vi "Mode_Select.vi"(1 "Input Data":T1) -> (0 "Signal Sequence [V]":dbl[](array[numeric]))   [LabVIEW 2023]
doc: "This Simple VI is aimed at extracting the sequece of interest, depending on the enumerator \"Type of the signal\".\nInputs:\n- Cluster (Matrix of the signals, Enumerator with the required type of signal).\nOutputs:\n- Required Signal"
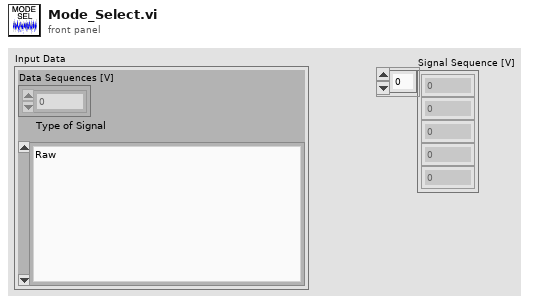
[diagram p1: front panel]
types:
  T1 = cluster{"Data Sequences [V]":dbl[][], "Type of Signal":enum16{"Raw", "Envelopped"}}
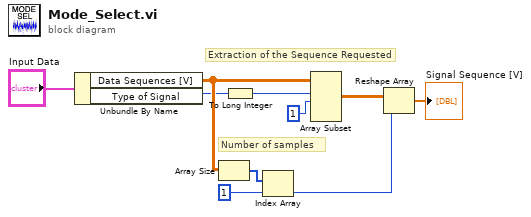
[diagram p0: block diagram]
diagram:
  # "Number of samples"
  # "Extraction of the Sequence Requested"
  n1 = Unbundle By Name("Input Data") -> ("Data Sequences [V]"=w3:dbl[][], "Type of Signal"=w1:enum16{"Raw", "Envelopped"})
  n2 = Array Size(array=w3) -> (size(s)=w5:i32[])
  n3 = To Long Integer(number=w1) -> (32bit integer=w8:i32)
  n4 = Index Array(array=w5, index=1) -> (element=w2:i32)
  n5 = Array Subset(array=w3, index (row)=w8, length (row)=1 ("length")) -> (w7:dbl[][])  [unwired: 2 in]
  n6 = Reshape Array(w7, w2) -> (→"Signal Sequence [V]":dbl[])
